vi "Modify_Cost_F()-1.vi"(3 "[IN] Additions to cost":i8, 4 "[IN] Current Index":i32, 5 "[IN] Cost function":i8[](array[numeric])) -> (2 "[OUT] Cost function":i8[](array[numeric]))   [LabVIEW 2013]
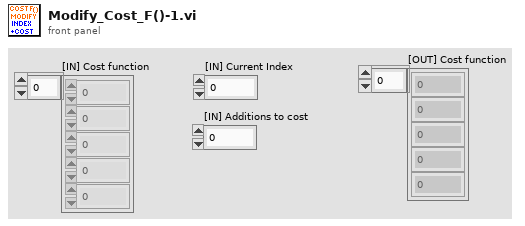
[diagram p1: front panel]
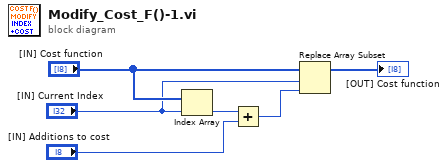
[diagram p0: block diagram]
diagram:
  n1 = Index Array(array="[IN] Cost function", index="[IN] Current Index") -> (element=w6:i8)
  n2 = Add(x=w6, y="[IN] Additions to cost") -> (x+y=w3:i8)
  n3 = Replace Array Subset(array="[IN] Cost function", new element=w3, index="[IN] Current Index") -> (→"[OUT] Cost function":i8[])
